vi "dependency-listorder-test.vi"(8 "error in (no error)":errorcluster) -> (0 "error out":errorcluster)   [LabVIEW 2013]
uses:
  _test-support-SMOs/SMO.TopLevel/Typedefs/Dependencies--Cluster.ctl
  _test-support-SMOs/SMO.A/SMO.A.lvclass
  _test-support-SMOs/SMO.TopLevel/SMO.TopLevel.lvclass
  <vilib>/addons/_JKI Toolkits/Caraya/classes/Test/Test.lvclass
  <vilib>/addons/_JKI Toolkits/Caraya/classes/Assert/Assert.lvclass
  src/SMO/SMO.lvclass
  <vilib>/Utility/VariantDataType/VariantType.lvlib
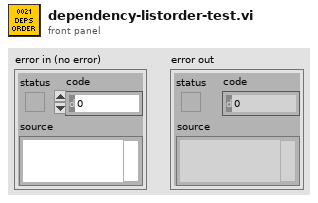
[diagram p1: front panel]
types:
  T1 = typedef "SMO.TopLevel.lvclass/Dependencies--Cluster.ctl" = cluster{"A":refnum<class "SMO.A.lvclass">, "A2":refnum<class "SMO.A.lvclass">, "A3":refnum<class "SMO.A.lvclass">, "A4":refnum<class "SMO.A.lvclass">}
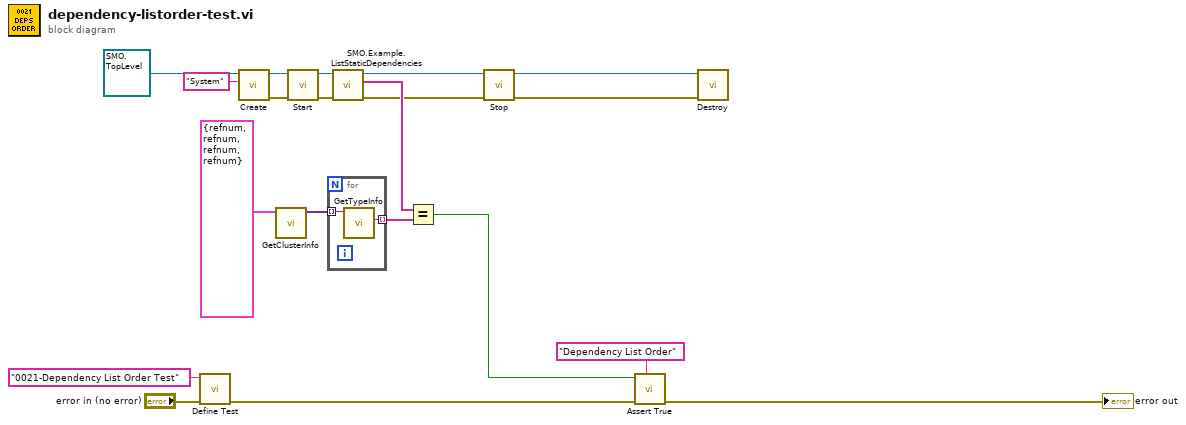
[diagram p0: block diagram]
diagram:
  n1 = call <vilib>:"Define Test.vi"("error in (no error)"="error in (no error)", "Label (VI Title)"="0021-Dependency List Order Test") -> ("error out"=w16:errorcluster)  [unwired: 9 in]
  n2 = call "Create.vi"("Subsystem Name (optional)"="System", "SMO"=refnum<class "SMO.TopLevel.lvclass"> refnum ("SMO.TopLevel.lvclass")) -> ("error out"=w6:errorcluster, "SMO out"=w8:refnum<class "SMO.TopLevel.lvclass">)  [unwired: 7 in, 1 out]
  n3 = call <vilib>:"GetClusterInfo.vi"("Variant"=T1 {"A"=refnum, "A2"=refnum, "A3"=refnum, "A4"=refnum} ("Dependencies")) -> ("Cluster Elements"=w12:variant[])  [unwired: 9 in, 1 out]
  n4 = call "Start.vi"("error in (no error)"=w6, "SMO"=w8) -> ("error out"=w5:errorcluster, "SMO out"=w7:refnum<class "SMO.TopLevel.lvclass">)  [unwired: 8 in]
  n5 = for {
    tunnel: w12 -> [w22] mode=indexing
    tunnel: [w21] -> w11 mode=indexing
    n6 = call <vilib>:"GetTypeInfo.vi"("Variant"=w22) -> ("Name"=w21:string)  [unwired: 6 in, 4 out]
  }
  n7 = call "SMO.Example.ListStaticDependencies.vi"("error in (no error)"=w5, "SMO.Example"=w7) -> ("error out"=w4:errorcluster, "Dependency Names"=w10:string[], "SMO.Example out"=w2:refnum<class "SMO.TopLevel.lvclass">)  [unwired: 7 in]
  n8 = Equal?(x=w10, y=w11) -> (x = y?=w9:bool)
  n9 = call "Stop.vi"("error in (no error)"=w4, "SMO"=w2) -> ("error out"=w3:errorcluster, "SMO out"=w1:refnum<class "SMO.TopLevel.lvclass">)  [unwired: 8 in]
  n10 = call <vilib>:"Assert True.vi"("Label"="Dependency List Order", "error in (no error)"=w16, "True?"=w9) -> ("error out"=→"error out":errorcluster)  [unwired: 8 in]
  n11 = call "Destroy.vi"("error in (no error)"=w3, "SMO"=w1) -> ()  [unwired: 9 in, 1 out]
